vi "LJM_eWriteName.vi"(0 "Handle In":i32, 5 "Name":string, 9 "Value":dbl format="%.2f", 11 "error in":errorcluster) -> (4 "Handle Out":i32, 15 "error out":errorcluster)   [LabVIEW 2025]
uses:
  labjackm.dll
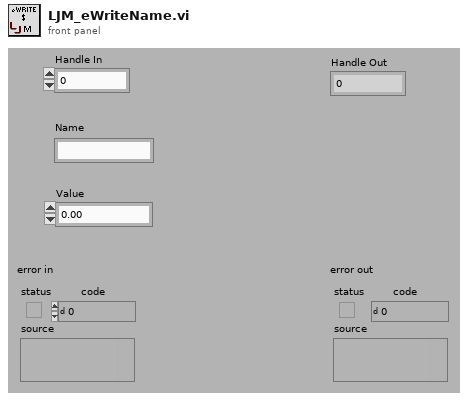
[diagram p1: front panel]
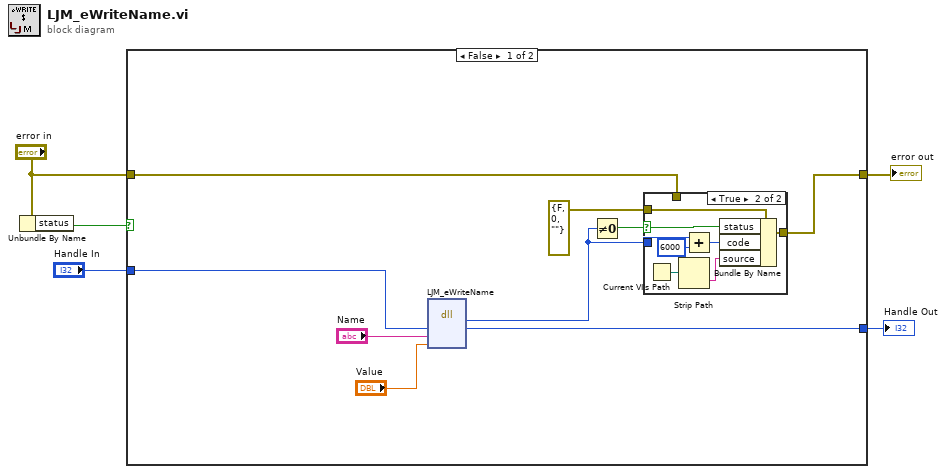
[diagram p0: block diagram]
diagram:
  n1 = Unbundle By Name("error in") -> ("status"=w5:bool)
  n2 = case shown="False" w5 {
    tunnel: "error in" -> [w8 w25]
    tunnel: [w11 w25] -> w3
    tunnel: [w7 w24] -> w2
    tunnel: "Handle In" -> [w6 w24]
    frame False {
      n3 = dll-call lib="labjackm.dll" fn="LJM_eWriteName"("Handle"=w6, "Name"="Name", "Value"="Value") -> (w14:i32, "Handle"=w7:i32)  [unwired: 5 in, 2 out]
      n4 = Not Equal To 0?(x=w14) -> (x != 0?=w13:bool)
      n5 = case shown="True" w13 {
        selector: w13 -> [_ w22]
        tunnel: [w15 w23] -> w11
        tunnel: errorcluster {"status"=FALSE, "code"=0, "source"=""} ("error IO") -> [_ w21]
        tunnel: w14 -> [_ w17]
        tunnel: w8 -> [w15 _]
        frame False {
        }
        frame True {
          n6 = Current VI's Path() -> (path=w19:path)
          n7 = Strip Path(path=w19) -> (name=w20:string)  [unwired: 1 out]
          n8 = Add(x=w17, y=6000) -> (x+y=w18:i32)
          n9 = Bundle By Name(cluster=w21, "status"=w22, "code"=w18, "source"=w20) -> (w23:errorcluster)
        }
      }
    }
    frame True {
    }
  }
  "error out" <- w3
  "Handle Out" <- w2
